vi "Sequence Commands.vi"(11 "queue in":refnum<queue>) -> ()   [LabVIEW 2023]
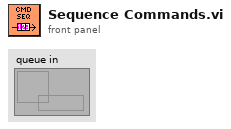
[diagram p1: front panel]
types:
  T1 = cluster{"Time (s)":dbl, "Command out":cluster{"Name":string, "vi reference":refnum<vi>, i32[], variant[]}}
  T2 = cluster{"Name":string, "vi reference":refnum<vi>, i32[], variant[]}
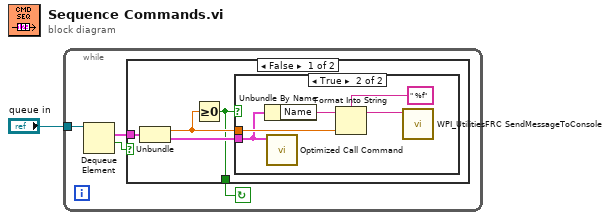
[diagram p0: block diagram]
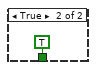
[diagram p3: hidden frame]
diagram:
  n1 = while {
    tunnel: "queue in" -> [w2]
    stop <- w3 continue-if-true
    n2 = Dequeue Element(queue=w2) -> (element=w5:T1, timed out?=w4:bool)  [unwired: 2 in, 2 out]
    n3 = case shown="False" w4 {
      tunnel: w5 -> [w9 _]
      tunnel: [w6 TRUE] -> w3
      frame False {
        n4 = Unbundle(w9) -> ("Time (s)"=w7:dbl, "Command out"=w8:T2)
        n5 = Greater Or Equal To 0?(x=w7) -> (x >= 0?=w6:bool)
        n6 = case shown="True" w6 {
          tunnel: w8 -> [_ w11]
          tunnel: w7 -> [_ w12]
          frame False {
          }
          frame True {
            n7 = Unbundle By Name(w11) -> ("Name"=w14:string)
            n8 = call "Optimized Call Command.vi"("Command"=w11) -> ()  [unwired: 10 in, 1 out]
            n9 = Format Into String(format string=" %f", initial string=w14, w12) -> (resulting string=w10:string)  [unwired: 1 in, 1 out]
            n10 = call <vilib>:"WPI_UtilitiesFRC SendMessageToConsole.vi"("Message"=w10) -> ()  [unwired: 14 in, 1 out]
          }
        }
      }
      frame True {
      }
    }
  }
